vi "re_run_task_lua.vi"(5 "LuaVIEW reference":T1) -> (15 "error out":errorcluster)   [LabVIEW 2012]
doc: "Call the \"Run Task\" Lua API VI to prepare, pre-process, and run a task script. This creates a seperate execution context in which the task will commence running asynchronously from the calling script. This function returns as soon as the task is finished initializing. Normally, this implies that the main script and any import scripts involved with the task could be properly loaded, compiled, and executed up to the main script. However it is possible for a task to perform deferred initialization using the \"--#defer\" preprocessor keyword. In that case this function will return without error only after the task has called the <code>task.initalized</code> function. This is useful when the started task needs to perform a series of error prone additional initialization actions or when the remainder of the launching script depends on resources initialized by the task being run.\n\nIf the task script is contained in a file, a relative path or bare filename will be resolved by searching relative to the configured script search directories. If no script search directories are configured, the resource base path is searched. If this function is called from a task context, the directory holding the main script of the calling task is searched first.\nParameters:\nstr:name, when the optional task script string is not specified, this is the filename plus any path from which to load the task script. Otherwise it is the name used to refer to the task script when reporting errors.\n[str:script], optional task script string allows direct specification of a bit of Lua code.\nResults:\nstr:identifier, identifier of the run task.\nErrors:\nCould not load task script or import script.\nError while preprrocessing task script or import script.\nCompilation error in task script or import script.\nTask identifier already in use.\nAny error thrown while initializing the task."
uses:
  typedefs/t_LuaVIEW Reference.ctl
  subvis/private/LuaVIEW Push (string).vi
  subvis/private/LuaVIEW Pull (path).vi
  subvis/private/LuaVIEW Pull (string).vi
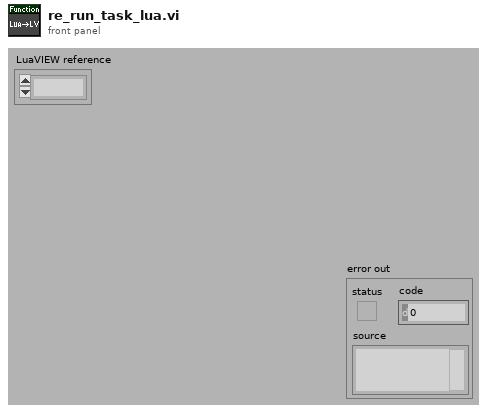
[diagram p1: front panel]
types:
  T1 = typedef "t_LuaVIEW Reference.ctl" = refnum<k1>
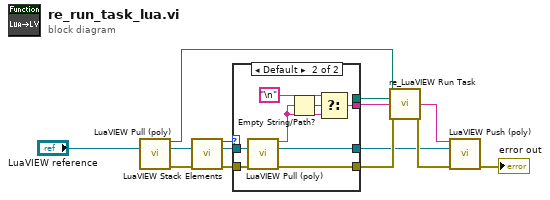
[diagram p0: block diagram]
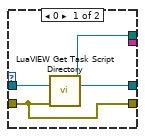
[diagram p2: hidden frame]
diagram:
  n1 = call-poly "LuaVIEW Pull (poly).vi"("LuaVIEW reference in"="LuaVIEW reference") -> ("path"=w1:path, "LuaVIEW reference out"=w12:T1, "error out"=w13:errorcluster)  [unwired: 12 in]
  n2 = call "LuaVIEW Stack Elements.vi"("LuaVIEW reference in"=w12, "error in (no error)"=w13) -> ("elements"=w11:i32, "LuaVIEW reference out"=w8:T1, "error out"=w10:errorcluster)  [unwired: 11 in]
  n3 = case shown="Default" w11 {
    tunnel: w10 -> [w18 w26]
    tunnel: [w18 w25] -> w6
    tunnel: [_ w24] -> w9
    tunnel: w8 -> [w15 w19]
    tunnel: [w16 w20] -> w3
    tunnel: [w17 _] -> w7
    frame 0 {
      n4 = call "LuaVIEW Get Task Script Directory.vi"("LuaVIEW reference in"=w15, "error in (no error)"=w18) -> ("task script directory"=w17:path, "LuaVIEW reference out"=w16:T1)  [unwired: 11 in, 1 out]
    }
    frame Default {
      n5 = call-poly "LuaVIEW Pull (poly).vi"("LuaVIEW reference in"=w19, "error in (no error)"=w26) -> ("string"=w22:string, "LuaVIEW reference out"=w20:T1, "error out"=w25:errorcluster)  [unwired: 11 in]
      n6 = Empty String/Path?(string/path=w22) -> (empty?=w23:bool)
      n7 = Select(t="\n", s=w23, f=w22) -> (s? t:f=w24:string)
    }
  }
  n8 = call "re_LuaVIEW Run Task.vi"("script file or name (no name)"=w1, "custom search directory (none)"=w7, "script string (\"\" == load from file)"=w9, "error in (no error)"=w6) -> ("identifier"=w4:string, "error out"=w5:errorcluster)  [unwired: 9 in, 1 out]
  n9 = call-poly "LuaVIEW Push (poly).vi"("string"=w4, "LuaVIEW reference in"=w3, "error in (no error)"=w5) -> ("error out"=→"error out":errorcluster)  [unwired: 11 in, 1 out]
